vi "picoquant_write_data_logger.vi"(8 "error in (no error)":errorcluster, 10 "data_logger.lvclass":refnum<class "data_logger.lvclass">, 11 "hydraharp in":refnum<class "hydraharp.lvclass">) -> (0 "error out":errorcluster, 3 "hydraharp out":refnum<class "hydraharp.lvclass">)   [LabVIEW 2015, in "hydraharp.lvclass"]
uses:
  hydraharp.lvclass
  Data Logger Class/data_logger.lvclass
  hydraharp.lvclass/hydraharp.ctl
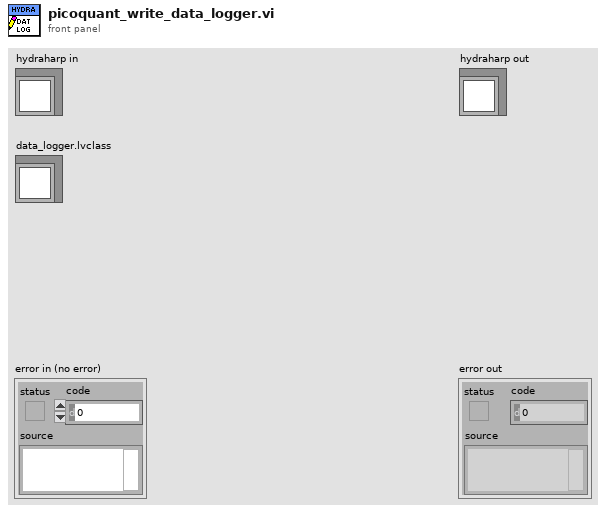
[diagram p1: front panel]
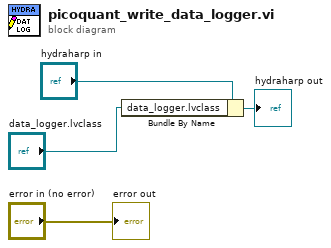
[diagram p0: block diagram]
diagram:
  n1 = Bundle By Name(cluster="hydraharp in", "data_logger.lvclass"="data_logger.lvclass") -> (→"hydraharp out":refnum<class "hydraharp.lvclass">)
  "error out" <- "error in (no error)"
